vi "Running.vi"(8 "error in (no error)":errorcluster, 11 "CIFTemplatePlugin in":refnum<class "CIFTemplatePlugin.lvclass">) -> (0 "error out":errorcluster, 2 "Destroy":bool, 3 "CIFTemplatePlugin out":refnum<class "CIFTemplatePlugin.lvclass">)   [LabVIEW 2021, in "CIFTemplatePlugin.lvclass"]
uses:
  CIFTemplatePlugin.lvclass
  D:/dev/CIF-LVCore/src/CIFCore/Class/CIFCorePlugin.lvclass
  CIFCore/Class/CIFCorePlugin.lvclass/CIFCorePlugin.ctl
  CIFTemplatePlugin.lvclass/CIFTemplatePlugin.ctl
  Channels/CIFChannelMng/CIFChannelMng.lvclass/CIFChannelMng.ctl
  Channels/CIFChannels/CIFChannels.lvclass/CIFChannels.ctl
  Channels/CIF_NIChn/Double/CIF_NIChn_Double.lvclass/CIF_NIChn_Double.ctl
  Channels/CIF_NIChn/NIChn/CIF_NIChn.lvclass/CIF_NIChn.ctl
  Channels/CIF_NIChn/U64/CIF_NIChn_U64.lvclass/CIF_NIChn_U64.ctl
  CIFUtilities/CIFOutOfBand/CIFOutOfBand.lvclass/CIFOutOfBand.ctl
  CIFCore/Class/Typedef/Energized States.ctl
  CIFCore/Class/Accessors/Timestamps/Write Sleep TS.vi
  CIFCore/Class/SubVIs/Sleep.vi
  Logic.vi
  CIFCore/Class/Accessors/Write Energized State.vi
  CIFCore/Class/SubVIs/Read Core OOB RX.vi
  gRPC/Read OOB RX.vi
  gRPC/Send OOB TX.vi
  CIFCore/OOB/OOB_Tx/Send/Update Status Command.vi
  CIFCore/OOB/OOB_Tx/Send/Update Override Command.vi
  CIFCore/Class/Accessors/Read Update Channel OOB.vi
  CIFCore/OOB/OOB_Tx/Send/Update Channel List Command.vi
  CIFCore/Class/Accessors/Read Channel Status.vi
  CIFCore/Class/Accessors/Write Update Channel OOB.vi
  CIFUtilities/CIFClocks/Core/Sleep Until Future Time.vi
  CIFUtilities/CIFClocks/Core/Get Time.vi
  CIFCore/Class/Accessors/Timestamps/Write Execute TS.vi
  <vilib>/Utility/error.llb/Clear Errors.vi
  CIFCore/Class/Accessors/Read Sleep Limits (ns).vi
  CIFCore/Class/Accessors/Timestamps/Write Target Wake TS.vi
  CIFCore/Common/Utilities/Add Error.vi
  CIFCore/Class/Accessors/Read Plugin Name.vi
  CIFCore/Class/Accessors/Get Time.vi
  CIFCore/Class/Accessors/Timestamps/Read Running TS.vi
  CIFCore/Class/Accessors/Read Running Internal Data.vi
  CIFCore/Class/Accessors/Read Timing Override.vi
  CIFCore/Class/Accessors/Read Common Config.vi
  Channels/CIF_NIChn/Double/Core/Read Double Direct Dispatch.vi
  Channels/CIF_NIChn/U64/Core/Read U64 Direct Dispatch.vi
  Channels/CIF_NIChn/Double/Core/Write Double Direct Dispatch.vi
  Channels/CIF_NIChn/U64/Core/Write U64 Direct Dispatch.vi
  CIFCore/Class/Accessors/Read Channel Array.vi
  CIFCore/Class/Accessors/Write Channel Array.vi
  CIFCore/Class/Accessors/Monitor/Write Double 1.vi
  CIFCore/Class/Accessors/Monitor/Write U64 1.vi
  CIFCore/Class/Accessors/Monitor/Write I64 1.vi
  CIFCore/Class/Accessors/Monitor/Write I64 2.vi
  CIFCore/Common/Utilities/Update Cycle Time.vi
  CIFCore/Common/Utilities/Update Delta Time.vi
  CIFCore/Class/Accessors/Timestamps/Write Housekeeping TS.vi
  CIFCore/Class/Benchmarking/Adjust Idle Benchmark.vi
  CIFCore/Class/Accessors/Timestamps/Read Execute TS.vi
  CIFCore/Class/Accessors/Timestamps/Read Housekeeping TS.vi
  CIFCore/Class/Accessors/Timestamps/Read Sleep TS.vi
  CIFCore/Class/Accessors/Timestamps/Read Target Wake TS.vi
  CIFCore/OOB/OOB_Rx/Receive/Check for OOB Commands.vi
  CIFCore/Class/SubVIs/Refresh Stats.vi
  OOB/OOB_Rx/Receive/Check for OOB Commands.vi
  OOB/OOB_Rx/Receive/Read Data.vi
  OOB/OOB_Tx/Send/Update Data.vi
  CIFCore/Class/Accessors/Read Refresh.vi
  CIFUtilities/CIFOutOfBand/Write OOB DVR.vi
  CIFUtilities/CIFOutOfBand/Utilities/Command to Bitwise Command.vi
  CIFUtilities/CIFOutOfBand/Accessors/Read Local OOB Data.vi
  CIFUtilities/CIFOutOfBand/Accessors/Write Local OOB Data.vi
  Channels/CIFChannelMng/Accessors/Read Update OOB.vi
  Channels/CIFChannelMng/Accessors/Read Channel Status for OOB.vi
  Channels/CIFChannelMng/Accessors/Write Update OOB.vi
  CIFUtilities/CIFClocks/Time Conversion/LabVIEW Time to UTC Time.vi
  CIFCore/Common/Utilities/Append Error Location.vi
  Channels/CIF_NIChn/NIChn/Accessors/Read CIF Channel.vi
  Channels/CIF_NIChn/NIChn/SubVIs/Check Disconnect.vi
  Channels/CIF_NIChn/Double/Core/Read Double Direct Dispatch.vi/cbead010-ab61-49ec-ac6c-083511305d37.vi
  Channels/CIF_NIChn/NIChn/Accessors/Write CIF Channel.vi
  Channels/CIFChannels/Accessors/Read Channel State.vi
  Channels/CIFChannels/Accessors/Read Direction.vi
  Channels/CIFChannels/Accessors/Read Forced.vi
  Channels/CIF_NIChn/U64/Core/Read U64 Direct Dispatch.vi/cbead010-ab61-49ec-ac6c-083511305d37.vi
  Channels/CIF_NIChn/Double/Core/Write Double Direct Dispatch.vi/e6e5dc56-0fe0-434b-816e-55c2e61471c2.vi
  Channels/CIF_NIChn/U64/Core/Write U64 Direct Dispatch.vi/e6e5dc56-0fe0-434b-816e-55c2e61471c2.vi
  Channels/CIFChannelMng/Accessors/Read Channel Array.vi
  Channels/CIFChannelMng/Accessors/Write Channel Array.vi
  CIFUtilities/CIFOutOfBand/Read OOB DVR.vi
  CIFCore/OOB/OOB_Rx/Private/Command Settings.vi
  OOB/OOB_Rx/Private/Command Settings.vi
  OOB/OOB_Rx/Private/Read Payload.vi
  Channels/CIFChannels/Accessors/Write Channel State.vi
  Channels/CIFChannels/Accessors/Read Disconnect Behavior.vi
  Channels/CIF_NIChn/Double/Core/Read Double Direct Dispatch.vi/cbead010-ab61-49ec-ac6c-083511305d37.vi/c28b0ead-42ad-4072-80a2-aca7f2bd7ce3.vi
  Channels/CIF_NIChn/Double/Core/Read Double Direct Dispatch.vi/cbead010-ab61-49ec-ac6c-083511305d37.vi/219d0231-d98b-4193-b5cc-84f90e3c9091.vi
  <vilib>/CIFChannels/SubVIs/Get dll Path.vi
  Channels/CIF_NIChn/U64/Core/Read U64 Direct Dispatch.vi/cbead010-ab61-49ec-ac6c-083511305d37.vi/c28b0ead-42ad-4072-80a2-aca7f2bd7ce3.vi
  Channels/CIF_NIChn/U64/Core/Read U64 Direct Dispatch.vi/cbead010-ab61-49ec-ac6c-083511305d37.vi/219d0231-d98b-4193-b5cc-84f90e3c9091.vi
  Channels/CIF_NIChn/Double/Core/Write Double Direct Dispatch.vi/e6e5dc56-0fe0-434b-816e-55c2e61471c2.vi/4bc1c15b-36ab-481f-b8dd-c64075ce723a.vi
  Channels/CIF_NIChn/Double/Core/Write Double Direct Dispatch.vi/e6e5dc56-0fe0-434b-816e-55c2e61471c2.vi/d83cb72b-7713-41fc-a3d1-682de79cf574.vi
  Channels/CIF_NIChn/U64/Core/Write U64 Direct Dispatch.vi/e6e5dc56-0fe0-434b-816e-55c2e61471c2.vi/4bc1c15b-36ab-481f-b8dd-c64075ce723a.vi
  Channels/CIF_NIChn/U64/Core/Write U64 Direct Dispatch.vi/e6e5dc56-0fe0-434b-816e-55c2e61471c2.vi/d83cb72b-7713-41fc-a3d1-682de79cf574.vi
  Channels/CIF_NIChn/Double/CIF_NIChn_Double.lvclass
  D:/dev/CIF-LVCore/src/Channels/CIFChannels/CIFChannels.lvclass
  D:/dev/CIF-LVCore/src/Channels/CIF_NIChn/NIChn/CIF_NIChnl.lvclass
  Channels/CIF_NIChn/NIChn/CIF_NIChn.lvclass
  Channels/CIF_NIChn/U64/CIF_NIChn_U64.lvclass
  OOB/OOB_Rx/CIFTCustomOOB_Rx.lvclass
  D:/dev/CIF-LVCore/src/CIFUtilities/CIFOutOfBand/CIFOutOfBand.lvclass
  OOB/OOB_Tx/CIFCustomOOB_Tx.lvclass
  CIFCore/OOB/OOB_Tx/CIFCoreOOB_Tx.lvclass
  CIFCore/OOB/OOB_Rx/CIFCoreOOB_Rx.lvclass
  CIFCore/Class/SubVIs/Channels/Connect Channels.vi
  CIFCore/Class/SubVIs/Channels/Force Channels.vi
  Channels/CIFChannels/CIFChannels.lvclass
  CIFCore/Class/CIFCorePlugin.lvclass
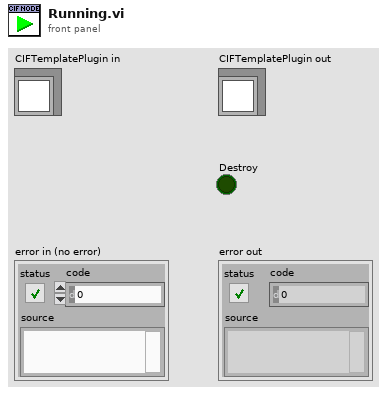
[diagram p1: front panel]
types:
  T1 = typedef "CIFCorePlugin.lvclass/Energized States.ctl" = enum16{"Listen", "Prepare", "Execute", "Housekeep", "Cleanup", "Destroy"}
  T2 = typedef "CIFCorePlugin.lvclass/Running State Logic.ctl" = enum16{"Execute", "Housekeep", "Cleanup", "Error", "Destroy"}
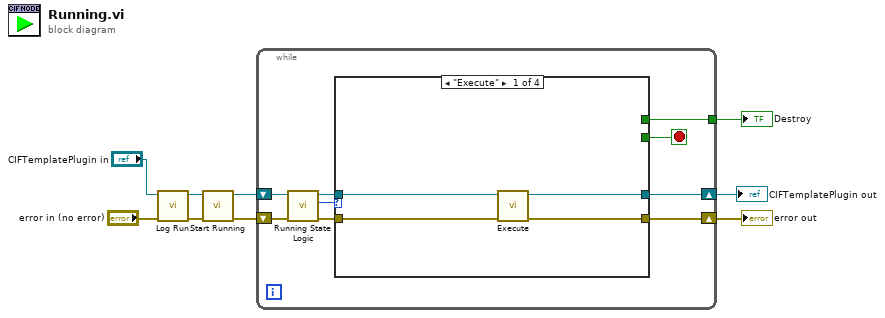
[diagram p0: block diagram]
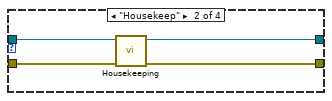
[diagram p2: hidden frame]
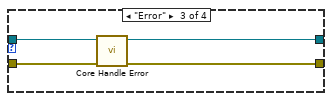
[diagram p3: hidden frame]
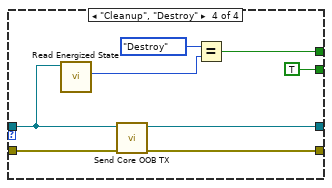
[diagram p4: hidden frame]
diagram:
  n1 = call "Log Run.vi"("error in (no error)"="error in (no error)", "CIFCorePlugin in"="CIFTemplatePlugin in") -> ("error out"=w4:errorcluster, "CIFCorePlugin out"=w3:refnum<class "CIFTemplatePlugin.lvclass">)  [unwired: 8 in]
  n2 = call "Start Running.vi"("error in (no error)"=w4, "CIFCorePlugin in"=w3) -> ("error out"=w6:errorcluster, "CIFCorePlugin out"=w7:refnum<class "CIFTemplatePlugin.lvclass">)  [unwired: 8 in]
  n3 = while {
    shift-right: [w13] -> w1
    shift-left: w7 -> [w18]
    shift-right: [w12] -> w8
    shift-left: w6 -> [w17]
    tunnel: [w10] -> w9
    stop <- w11 stop-if-true
    n4 = call "Running State Logic.vi"("error in (no error)"=w17, "CIFCorePlugin in"=w18) -> ("error out"=w14:errorcluster, "Running State Logic"=w16:T2, "CIFCorePlugin out"=w15:refnum<class "CIFTemplatePlugin.lvclass">)  [unwired: 7 in]
    n5 = case shown="\"Execute\"" w16 {
      tunnel: w15 -> [w22 w26 w30 w32]
      tunnel: w14 -> [w21 w25 w29 w37]
      tunnel: [w20 w24 w28 w36] -> w13
      tunnel: [w19 w23 w27 w35] -> w12
      tunnel: [_ _ _ TRUE] -> w11
      tunnel: [_ _ _ w33] -> w10
      frame "Execute" {
        n6 = call "Execute.vi"("error in (no error)"=w21, "CIFTemplatePlugin in"=w22) -> ("error out"=w19:errorcluster, "CIFTemplatePlugin out"=w20:refnum<class "CIFTemplatePlugin.lvclass">)  [unwired: 8 in]
      }
      frame "Housekeep" {
        n7 = call "Housekeeping.vi"("error in (no error)"=w25, "CIFTemplatePlugin in"=w26) -> ("error out"=w23:errorcluster, "CIFTemplatePlugin out"=w24:refnum<class "CIFTemplatePlugin.lvclass">)  [unwired: 8 in]
      }
      frame "Error" {
        n8 = call "Core Handle Error.vi"("error in (no error)"=w29, "CIFTemplateNode in"=w30) -> ("error out"=w27:errorcluster, "CIFTemplateNode out"=w28:refnum<class "CIFTemplatePlugin.lvclass">)  [unwired: 8 in]
      }
      frame "Cleanup", "Destroy" {
        n9 = call "Read Energized State.vi"("CIFCorePlugin in"=w32) -> ("Energized State"=w31:T1)  [unwired: 8 in, 2 out]
        n10 = call "Send Core OOB TX.vi"("error in (no error)"=w37, "CIFCorePlugin in"=w32) -> ("error out"=w35:errorcluster, "CIFCorePlugin out"=w36:refnum<class "CIFTemplatePlugin.lvclass">)  [unwired: 8 in]
        n11 = Equal?(x=Energized_States."Destroy", y=w31) -> (x = y?=w33:bool)
      }
    }
  }
  "error out" <- w8
  "Destroy" <- w9
  "CIFTemplatePlugin out" <- w1
